vi "rs3 Advanced set A-factor.vi"(8 "error in (no error)":errorcluster, 10 "A-factor (0-0.2)":sgl, 11 "device in":u64) -> (0 "error out":errorcluster, 1 "error":u64, 3 "Dev out":u64)   [LabVIEW 2017, in "libRealSense3.lvlib"]
doc: "Sets the A-factor that can improve the depth linearity."
uses:
  libRealSense3.lvlib
  realsense2.dll
panel:
  # "RS3 Adv. Set A-factor"
  # "(C) 2020 Intel Corp.,  AGJ"
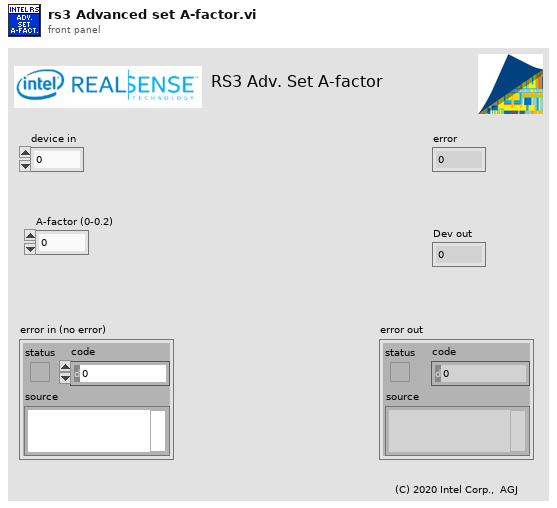
[diagram p1: front panel]
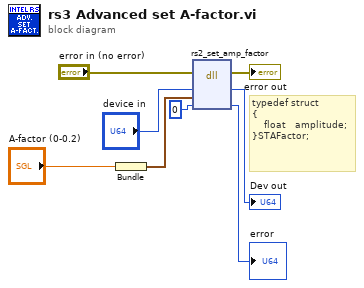
[diagram p0: block diagram]
diagram:
  # "typedef struct\n{\n    float   amplitude;\n}STAFactor;"
  n1 = Bundle("A-factor (0-0.2)"="A-factor (0-0.2)") -> (w1:cluster{"A-factor (0-0.2)":sgl})  [unwired: 1 in]
  n2 = dll-call lib="C:/Users/agrunnet/Documents/libRealSense6/realsense2.dll" fn="rs2_set_amp_factor"(error in="error in (no error)", "device"="device in", "A-factor"=w1, "error"=u64 0) -> (error out=→"error out":errorcluster, "device"=→"Dev out":u64, "error"=→"error":u64)  [unwired: 4 in, 1 out]
